vi "Read Colors.vi"(9 "Boolean in":refnum<class "Boolean.lvclass">) -> (3 "Boolean out":refnum<class "Boolean.lvclass">, 4 "Colors":cluster{u32, u32}[](array[cluster]))   [LabVIEW 2014, in "Boolean.lvclass"]
uses:
  Boolean.lvclass
  Boolean.lvclass/Boolean.ctl
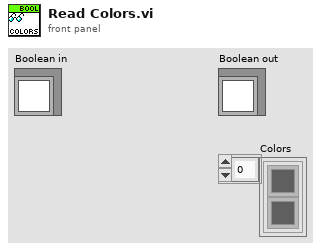
[diagram p1: front panel]
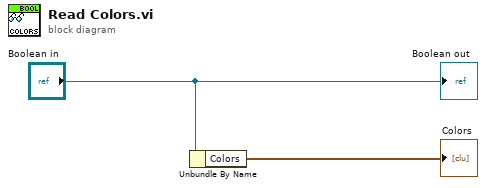
[diagram p0: block diagram]
diagram:
  n1 = Unbundle By Name("Boolean in") -> ("Colors"=→"Colors":cluster{u32, u32}[])
  "Boolean out" <- "Boolean in"
